vi "createSeqFileFromData.vi"(10 "Sequence File Data":T1[](array[typedef]), 11 "Sequence Context In":refnum<k7>) -> (0 "error out":errorcluster, 3 "NewSequenceFile":refnum<k7>)   [LabVIEW 2011]
doc: "This VI demonstrates how to cast a SequenceFile object in order access properties of the PropertyObjectFile and PropertyObject parent classes"
uses:
  Common/ReadStepsFromFile.llb/ReadStepsFromFile - SequenceData.ctl
  Common/ReadStepsFromFile.llb/ReadStepsFromFile - StepGroup.ctl
  Common/ReadStepsFromFile.llb/ReadStepsFromFile - StepData.ctl
  Common/ReadStepsFromFile.llb/ReadStepsFromFile - StepProperties.ctl
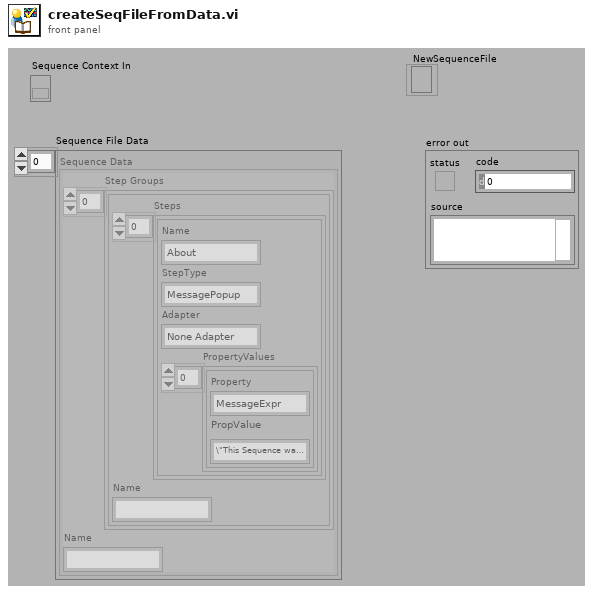
[diagram p1: front panel]
types:
  T1 = typedef "ReadStepsFromFile - SequenceData.ctl" = cluster{"Step Groups":T2[], "Name":string}
  T2 = typedef "ReadStepsFromFile - StepGroup.ctl" = cluster{"Steps":T3[], "Name":string}
  T3 = typedef "ReadStepsFromFile - StepData.ctl" = cluster{"Name":string, "StepType":string, "Adapter":string, "PropertyValues":T4[]}
  T4 = typedef "ReadStepsFromFile - StepProperties.ctl" = cluster{"Property":string, "PropValue":string}
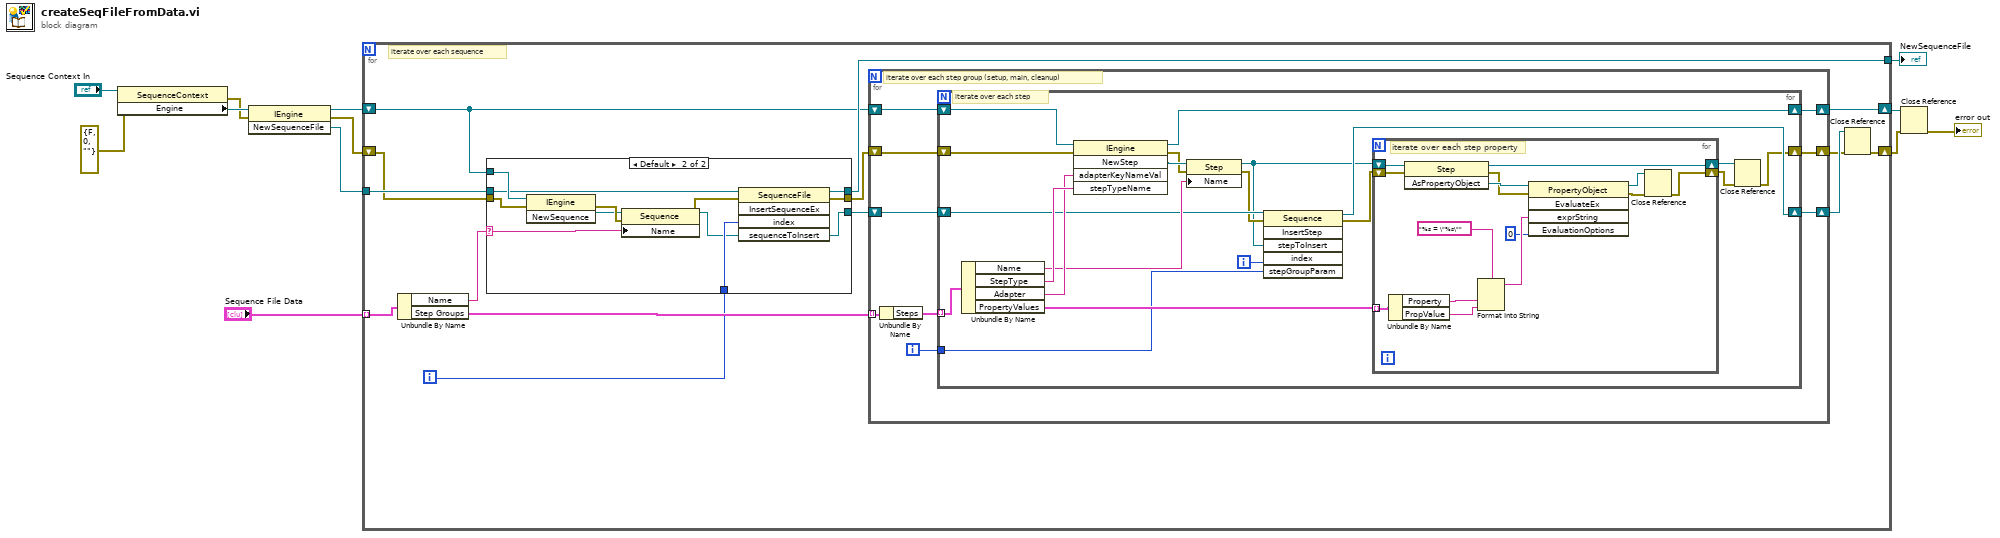
[diagram p0: block diagram]
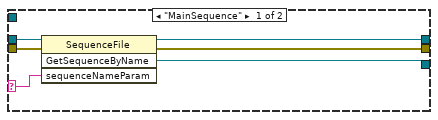
[diagram p2: hidden frame]
diagram:
  n1 = property class="SequenceContext"(reference="Sequence Context In", error in=errorcluster {"status"=FALSE, "code"=0, "source"=""} ("error in (no error)")) -> (error out=w3:errorcluster, "Engine"=w12:refnum<k7>)  [unwired: 1 out]
  n2 = invoke class="IEngine" method="NewSequenceFile"(reference=w12, error in=w3) -> (reference out=w10:refnum<k7>, error out=w8:errorcluster, "NewSequenceFile"=w11:refnum<k7>)  [unwired: 1 in]
  n3 = for {
    tunnel: "Sequence File Data" -> [w26] mode=indexing
    tunnel: w11 -> [w17]
    shift-right: [w22] -> w6
    shift-left: w8 -> [w16]
    tunnel: [w15] -> w7
    shift-right: [w13] -> w4
    shift-left: w10 -> [w14]
    i -> [w21]
    # "iterate over each sequence"
    n4 = Unbundle By Name(w26) -> ("Name"=w18:string, "Step Groups"=w25:T2[])
    n5 = case shown="Default" w18 {
      selector: w18 -> [w30 w39]
      tunnel: w16 -> [w32 w38]
      tunnel: w21 -> [_ w43]
      tunnel: w17 -> [w31 w33]
      tunnel: [w28 w42] -> w20
      tunnel: [w29 w40] -> w19
      tunnel: [w27 w35] -> w15
      tunnel: w14 -> [_ w34]
      frame "MainSequence" {
        n6 = invoke class="SequenceFile" method="GetSequenceByName"(reference=w31, error in=w32, "sequenceNameParam"=w30) -> (reference out=w27:refnum<k7>, error out=w28:errorcluster, "GetSequenceByName"=w29:refnum<k7>)  [unwired: 1 in, 1 out]
      }
      frame Default {
        n7 = invoke class="IEngine" method="NewSequence"(reference=w34, error in=w38) -> (error out=w37:errorcluster, "NewSequence"=w36:refnum<k7>)  [unwired: 1 in, 1 out]
        n8 = property class="Sequence"(reference=w36, error in=w37, "Name"=w39) -> (reference out=w40:refnum<k7>, error out=w41:errorcluster)
        n9 = invoke class="SequenceFile" method="InsertSequenceEx"(reference=w33, error in=w41, "index"=w43, "sequenceToInsert"=w40) -> (reference out=w35:refnum<k7>, error out=w42:errorcluster)  [unwired: 1 in, 3 out]
      }
    }
    n10 = for {
      tunnel: w25 -> [w51] mode=indexing
      shift-right: [w45] -> w23
      shift-left: w20 -> [w48]
      shift-right: [w44] -> w13
      shift-left: w14 -> [w52]
      shift-right: [w46] -> w24
      shift-left: w19 -> [w49]
      i -> [w47]
      # "iterate over each step group (setup, main, cleanup)"
      n11 = Unbundle By Name(w51) -> ("Steps"=w50:T3[])
      n12 = for {
        tunnel: w50 -> [w71] mode=indexing
        tunnel: w47 -> [w61]
        shift-right: [w59] -> w45
        shift-left: w48 -> [w63]
        shift-right: [w53] -> w44
        shift-left: w52 -> [w72]
        shift-right: [w60] -> w46
        shift-left: w49 -> [w64]
        i -> [w62]
        # "iterate over each step"
        n13 = Unbundle By Name(w71) -> ("Name"=w66:string, "StepType"=w70:string, "Adapter"=w69:string, "PropertyValues"=w65:T4[])
        n14 = invoke class="IEngine" method="NewStep"(reference=w72, error in=w63, "adapterKeyNameVal"=w69, "stepTypeName"=w70) -> (reference out=w53:refnum<k7>, error out=w67:errorcluster, "NewStep"=w68:refnum<k7>)  [unwired: 1 in, 2 out]
        n15 = property class="Step"(reference=w68, error in=w67, "Name"=w66) -> (reference out=w56:refnum<k7>, error out=w57:errorcluster)
        n16 = invoke class="Sequence" method="InsertStep"(reference=w64, error in=w57, "stepToInsert"=w56, "index"=w62, "stepGroupParam"=w61) -> (reference out=w60:refnum<k7>, error out=w58:errorcluster)  [unwired: 1 in, 4 out]
        n17 = for {
          tunnel: w65 -> [w86] mode=indexing
          shift-right: [w74] -> w55
          shift-left: w58 -> [w85]
          shift-right: [w75] -> w54
          shift-left: w56 -> [w73]
          # "iterate over each step property"
          n18 = Unbundle By Name(w86) -> ("Property"=w81:string, "PropValue"=w80:string)
          n19 = invoke class="Step" method="AsPropertyObject"(reference=w73, error in=w85) -> (reference out=w75:refnum<k7>, error out=w83:errorcluster, "AsPropertyObject"=w84:refnum<k7>)  [unwired: 1 in]
          n20 = Format Into String(format string="%s = \"%s\"", w81, w80) -> (resulting string=w79:string)  [unwired: 2 in, 1 out]
          n21 = invoke class="PropertyObject" method="EvaluateEx"(reference=w84, error in=w83, "exprString"=w79, "EvaluationOptions"=0) -> (reference out=w76:refnum<k7>, error out=w77:errorcluster)  [unwired: 1 in, 3 out]
          n22 = Close Reference(reference=w76, error in (no error)=w77) -> (error out=w74:errorcluster)
        }
        n23 = Close Reference(reference=w54, error in (no error)=w55) -> (error out=w59:errorcluster)
      }
    }
    n24 = Close Reference(reference=w24, error in (no error)=w23) -> (error out=w22:errorcluster)
  }
  "NewSequenceFile" <- w7
  n25 = Close Reference(reference=w4, error in (no error)=w6) -> (error out=→"error out":errorcluster)
